vi "MCL Number Of Current Handles.vi"() -> (3 "function return":i32)   [LabVIEW 2017, in "Madlib.lvlib"]
doc: "MADLIB_API int MCL_NumberOfCurrentHandles();"
uses:
  Madlib.lvlib
  Madlib.dll
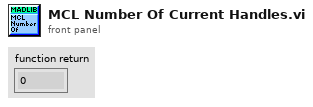
[diagram p1: front panel]
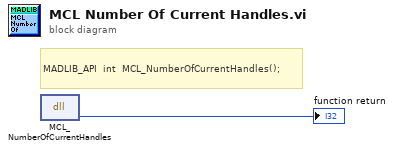
[diagram p0: block diagram]
diagram:
  # "MADLIB_API  int\t\tMCL_NumberOfCurrentHandles();"
  n1 = dll-call lib="C:/Users/francesco/dev/pump-probe/Piezo/lvlib/Madlib.*" fn="MCL_NumberOfCurrentHandles"() -> (→"function return":i32)  [unwired: 3 in, 2 out]
